vi "timer testing I dont like it.vi"   [LabVIEW 2018]
types:
  T1 = enum16{"Start Timer", "Get Time", "Pause", "Unpause"}
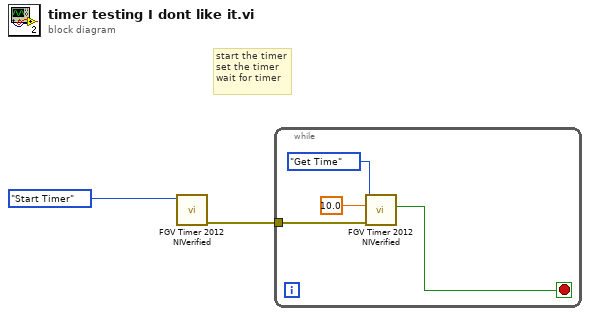
[diagram p0: block diagram]
diagram:
  # "start the timer\nset the timer\nwait for timer"
  n1 = call "FGV Timer 2012 NIVerified.vi"("Enum"=T1."Start Timer") -> ("error out"=w2:errorcluster)  [unwired: 7 in, 3 out]
  n2 = while {
    tunnel: w2 -> [w5]
    stop <- w6 stop-if-true
    n3 = call "FGV Timer 2012 NIVerified.vi"("error in (no error)"=w5, "Target Time (sec)"=10.0, "Enum"=T1."Get Time") -> ("Time Elapsed?"=w6:bool)  [unwired: 5 in, 3 out]
  }
